vi "new project.vi"(10 "Basic Inputs":T3={"Q.Plant"=0.0, "C.CoagDoseMax"=0.0, "C.CoagStock"=0.0, "Ti.CoagStock"=0.0, "EN.DrillSeries"=enum."English", "EN.TubeSeries"=enum."English", "N.SedTanks"=0.0, "N.SedBaysEst"=0.0, "W.SedPlate"=0.0, "L.SedPlateSheet"=0.0, "T.SedPlate"=0.0, "T.PlantWall"=0.03, "H.FlocOption"=0.01, "T.FlocBaffleRigidH"=0.03, "T.ConcreteMin"=0.3, "T.SedWeir"=0.3, "T.FlocBaffleRigidV"=108000.0} caption="Datos basicos" {"T.FlocBaffleRigidV" min=0.0 max=0.2 step=0.001 format="%#.1f"; "T.SedWeir" min=0.001 max=0.2 step=0.001 format="%#.1f"; "T.SedPlate" min=0.001 max=0.05 step=0.001 format="%#.1f"; "T.FlocBaffleRigidH" min=0.0 max=0.2 step=0.001 format="%#.1f"; "T.ConcreteMin" min=0.005 max=0.2 step=0.001 format="%#.1f"; "L.SedPlateSheet" min=0.3 max=8.0 step=0.01 format="%#.1f"; "N.SedBaysEst" min=1.0 max=20.0 step=1.0 format="%#.0f"; "N.SedTanks" min=1.0 max=20.0 step=1.0 format="%#.0f"; "Ti.CoagStock" min=43200.0 max=360000.0 step=3600.0 format="%#.1f"; "H.FlocOption" min=0.5 max=4.0 step=0.01 format="%#.2f"; "C.CoagStock" min=50.0 max=500.0 step=1.0 format="%#.0f"; "C.CoagDoseMax" min=0.03 max=0.2 step=0.005 format="%#.0f"; "Q.Plant" min=0.001 max=0.2 step=0.0001 format="%#.1f"; "T.PlantWall" min=0.05 max=0.5 step=0.001 format="%#.1f"; "W.SedPlate" min=0.5 max=3.0 step=0.001 format="%#.1f"}, 11 "Project Info":T1 caption="Información del proyecto") -> (0 "canceled":bool, 2 "Design Inputs out":T3={"Q.Plant"=0.0, "C.CoagDoseMax"=0.0, "C.CoagStock"=0.0, "Ti.CoagStock"=0.0, "EN.DrillSeries"=enum."English", "EN.TubeSeries"=enum."English", "N.SedTanks"=0.0, "N.SedBaysEst"=0.0, "W.SedPlate"=0.0, "L.SedPlateSheet"=0.0, "T.SedPlate"=0.0, "T.PlantWall"=0.03, "H.FlocOption"=0.01, "T.FlocBaffleRigidH"=0.03, "T.ConcreteMin"=0.3, "T.SedWeir"=0.3, "T.FlocBaffleRigidV"=108000.0} caption="Datos basicos" {"T.FlocBaffleRigidV" min=0.0 max=0.2 step=0.001 format="%#.1f"; "T.SedWeir" min=0.001 max=0.2 step=0.001 format="%#.1f"; "T.SedPlate" min=0.001 max=0.05 step=0.001 format="%#.1f"; "T.FlocBaffleRigidH" min=0.0 max=0.2 step=0.001 format="%#.1f"; "T.ConcreteMin" min=0.005 max=0.2 step=0.001 format="%#.1f"; "L.SedPlateSheet" min=0.3 max=8.0 step=0.01 format="%#.1f"; "N.SedBaysEst" min=1.0 max=20.0 step=1.0 format="%#.0f"; "N.SedTanks" min=1.0 max=20.0 step=1.0 format="%#.0f"; "Ti.CoagStock" min=43200.0 max=360000.0 step=3600.0 format="%#.1f"; "H.FlocOption" min=0.5 max=4.0 step=0.01 format="%#.2f"; "C.CoagStock" min=50.0 max=500.0 step=1.0 format="%#.0f"; "C.CoagDoseMax" min=0.03 max=0.2 step=0.005 format="%#.0f"; "Q.Plant" min=0.001 max=0.2 step=0.0001 format="%#.1f"; "T.PlantWall" min=0.05 max=0.5 step=0.001 format="%#.1f"; "W.SedPlate" min=0.5 max=3.0 step=0.001 format="%#.1f"}, 3 "Project Info out":T1 caption="Datos basicos")   [LabVIEW 2015]
uses:
  Project inputs.ctl
  Basic Inputs.ctl
  AguaClara Library.lvlib
panel:
  in  "Reset to Default":bool caption="Restablecer valores predeterminados"
  out "Design Inputs Label":string caption="Datos basicos"
  out "Project Info label":string caption="Información del proyecto"
  in  "Tab Control":enum32{" ", "  "}(tab) caption="Control de etiqueta"
  in  "Floc tank depth controls":T2={"HW.FlocEnd"=enum."User specified depth", "HW.FlocEndDepth"=2.0} caption="Opciones para la profundidad del floculador" {"HW.FlocEndDepth" min=0.5 max=5.0 step=0.01 format="%.2f"}
  in  "Cancel Button":bool caption="Cancelar"
  in  "OK Button":bool
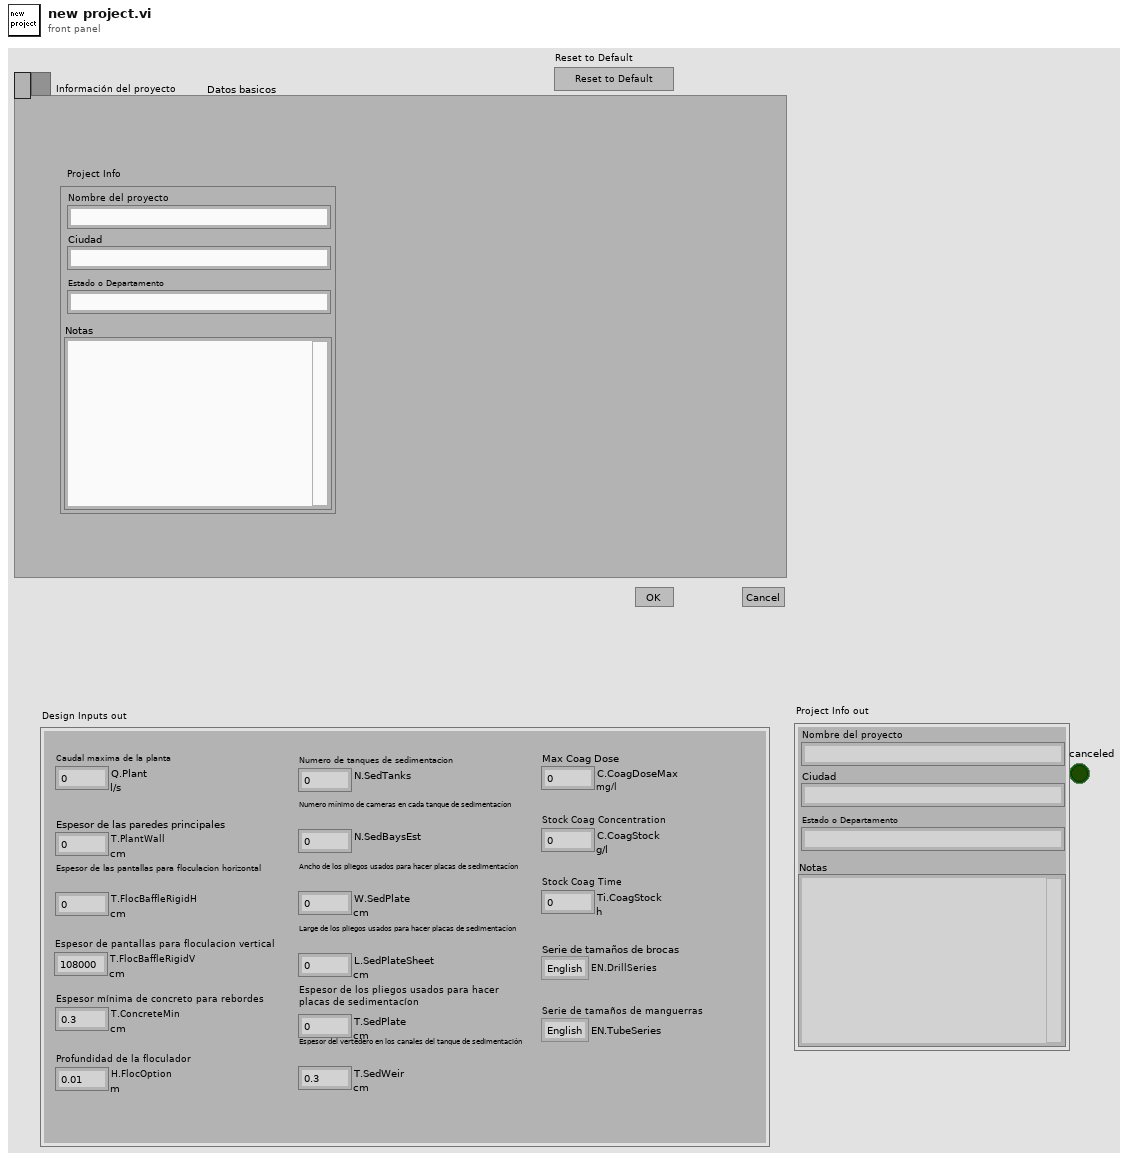
[diagram p1: front panel]
types:
  T1 = typedef "AguaClara Library.lvlib/Project inputs.ctl" = cluster{"Project Name":string, "City":string, "State":string, "Notes":string}
  T2 = cluster{"HW.FlocEnd":enum32{"User specified depth", "Same depth as sed tank", "Maximum depth for horizontal flow flocculator"}, "HW.FlocEndDepth":dbl[unit]}
  T3 = typedef "AguaClara Library.lvlib/Basic Inputs.ctl" = cluster{"Q.Plant":dbl[unit], "C.CoagDoseMax":dbl[unit], "C.CoagStock":dbl[unit], "Ti.CoagStock":dbl[unit], "EN.DrillSeries":enum16{"English", "Metric"}, "EN.TubeSeries":enum16{"English", "Metric"}, "N.SedTanks":dbl, "N.SedBaysEst":dbl, "W.SedPlate":dbl[unit], "L.SedPlateSheet":dbl[unit], "T.SedPlate":dbl[unit], "T.PlantWall":dbl[unit], "H.FlocOption":dbl[unit], "T.FlocBaffleRigidH":dbl[unit], "T.ConcreteMin":dbl[unit], "T.SedWeir":dbl[unit], "T.FlocBaffleRigidV":dbl[unit]}
  T4 = enum16{"load GUI", "write to GUI", "Update GUI", "write to basic inputs", "read from basic inputs"}
  T5 = typedef "Input Cluster.ctl" = cluster{"Project Info":T1, "Basic Inputs":T3}
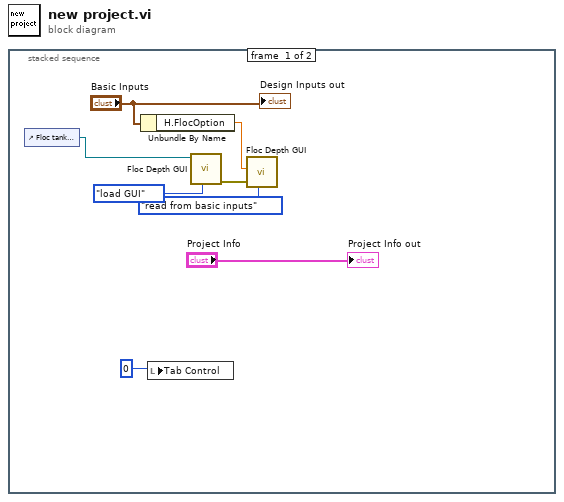
[diagram p0: block diagram]
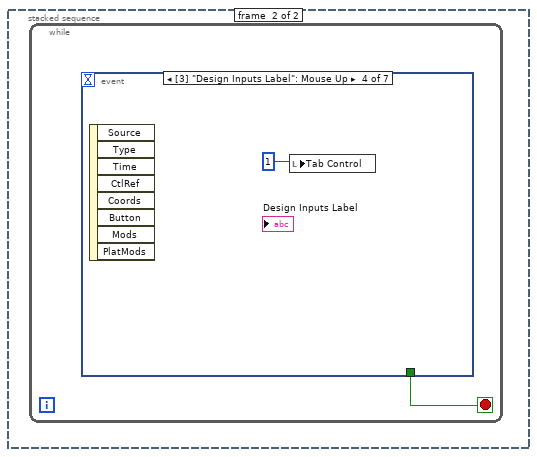
[diagram p2: hidden frame]
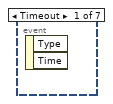
[diagram p3: hidden frame]
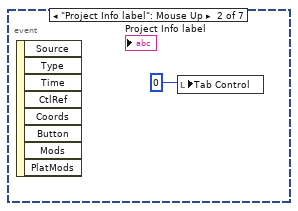
[diagram p4: hidden frame]
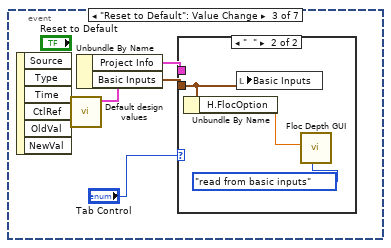
[diagram p5: hidden frame]
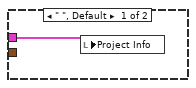
[diagram p6: hidden frame]
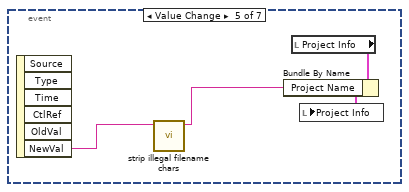
[diagram p7: hidden frame]
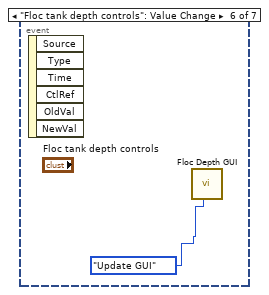
[diagram p8: hidden frame]
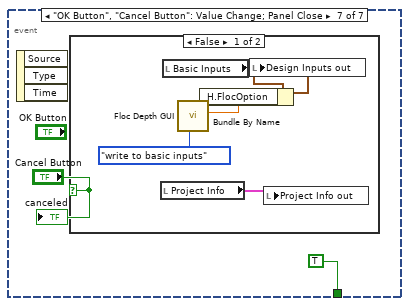
[diagram p9: hidden frame]
diagram:
  n1 = stacked-sequence {
    frame #0 {
      n2 = control-ref of="Floc tank depth controls"() -> (w2:refnum<vi>)
      n3 = Unbundle By Name("Basic Inputs") -> ("H.FlocOption"=w6:dbl[unit])
      n4 = local write "Tab Control"(0) -> ()
      n5 = call "Floc Depth GUI.vi"("Floc Depth r/w control"=T4."load GUI", "Floc Depth Ref 2"=w2) -> ("error out"=w5:errorcluster)  [unwired: 8 in, 1 out]
      n6 = call "Floc Depth GUI.vi"("Floc Depth r/w control"=T4."read from basic inputs", "error in (no error)"=w5, "HW.FlocEndDepthIntput"=w6) -> ()  [unwired: 7 in, 2 out]
      "Design Inputs out" <- "Basic Inputs"
      "Project Info out" <- "Project Info"
    }
    frame #1 {
      n7 = while {
        stop <- w9 stop-if-true
        n8 = event shown="[3] \"Design Inputs Label\": Mouse Up" {
          selector: _ -> [_ _ _ _ _ _ _]
          dyn-events: _ -> [_ _ _ _ _ _ _]
          timeout: _ -> [_ _ _ _ _ _ _]
          tunnel: [_ _ _ _ _ _ TRUE] -> w9
          event Timeout {
            n9 = event-data() -> ()  [unwired: 1 in, 2 out]
          }
          event "Project Info label": Mouse Up {
            n10 = event-data() -> ()  [unwired: 1 in, 8 out]
            n11 = local write "Tab Control"(0) -> ()
          }
          event "Reset to Default": Value Change {
            n12 = event-data() -> ()  [unwired: 1 in, 6 out]
            n13 = call "Default design values.vi"() -> ("Input Cluster"=w13:T5)  [unwired: 9 in, 2 out]
            n14 = Unbundle By Name(w13) -> ("Project Info"=w11:T1, "Basic Inputs"=w12:T3)
            n15 = case shown="\"  \"" "Tab Control" {
              tunnel: w12 -> [_ w18]
              tunnel: w11 -> [w15 _]
              frame " ", Default {
                n16 = local write "Project Info"(w15) -> ()
              }
              frame "  " {
                n17 = Unbundle By Name(w18) -> ("H.FlocOption"=w17:dbl[unit])
                n18 = local write "Basic Inputs"(w18) -> ()
                n19 = call "Floc Depth GUI.vi"("Floc Depth r/w control"=T4."read from basic inputs", "HW.FlocEndDepthIntput"=w17) -> ()  [unwired: 8 in, 2 out]
              }
            }
          }
          event "Design Inputs Label": Mouse Up {
            n20 = event-data() -> ()  [unwired: 1 in, 8 out]
            n21 = local write "Tab Control"(1) -> ()
          }
          event Value Change {
            n22 = event-data() -> ("NewVal"=w23:string)  [unwired: 1 in, 5 out]
            n23 = call "strip illegal filename chars.vi"("string in"=w23) -> ("string out"=w20:string)  [unwired: 10 in]
            n24 = local read "Project Info"() -> (w22:T1)
            n25 = Bundle By Name(cluster=w22, "Project Name"=w20) -> (w21:T1)
            n26 = local write "Project Info"(w21) -> ()
          }
          event "Floc tank depth controls": Value Change {
            n27 = event-data() -> ()  [unwired: 1 in, 6 out]
            n28 = call "Floc Depth GUI.vi"("Floc Depth r/w control"=T4."Update GUI") -> ()  [unwired: 9 in, 2 out]
          }
          event "OK Button", "Cancel Button": Value Change; Panel Close {
            n29 = event-data() -> ()  [unwired: 1 in, 3 out]
            n30 = case shown="False" "Cancel Button" {
              frame False {
                n31 = local read "Project Info"() -> (w31:T1)
                n32 = local read "Basic Inputs"() -> (w30:T3)
                n33 = call "Floc Depth GUI.vi"("Floc Depth r/w control"=T4."write to basic inputs") -> ("HW.FlocEndDepth Output"=w28:dbl[unit])  [unwired: 9 in, 1 out]
                n34 = Bundle By Name(cluster=w30, "H.FlocOption"=w28) -> (w29:T3)
                n35 = local write "Design Inputs out"(w29) -> ()
                n36 = local write "Project Info out"(w31) -> ()
              }
              frame True {
              }
            }
            "canceled" <- "Cancel Button"
          }
        }
      }
    }
  }
